vi "Instrument fgv.vi"(7 "Enum":T1(ring), 8 "error in (no error) 2":errorcluster, 10 "WriteCC1":string[](array[string])=[""], 11 "INPUT":T2) -> (0 "error":errorcluster, 2 "WriteCC1 2":string[](array[string]), 3 "output":T2)   [LabVIEW 2025]
uses:
  <vilib>/Instr/_visa.llb/VISA Configure Serial Port (Instr).vi
panel:
  out "error out":errorcluster
  out "Serial Settings:Number of Bytes at Serial Port":u32
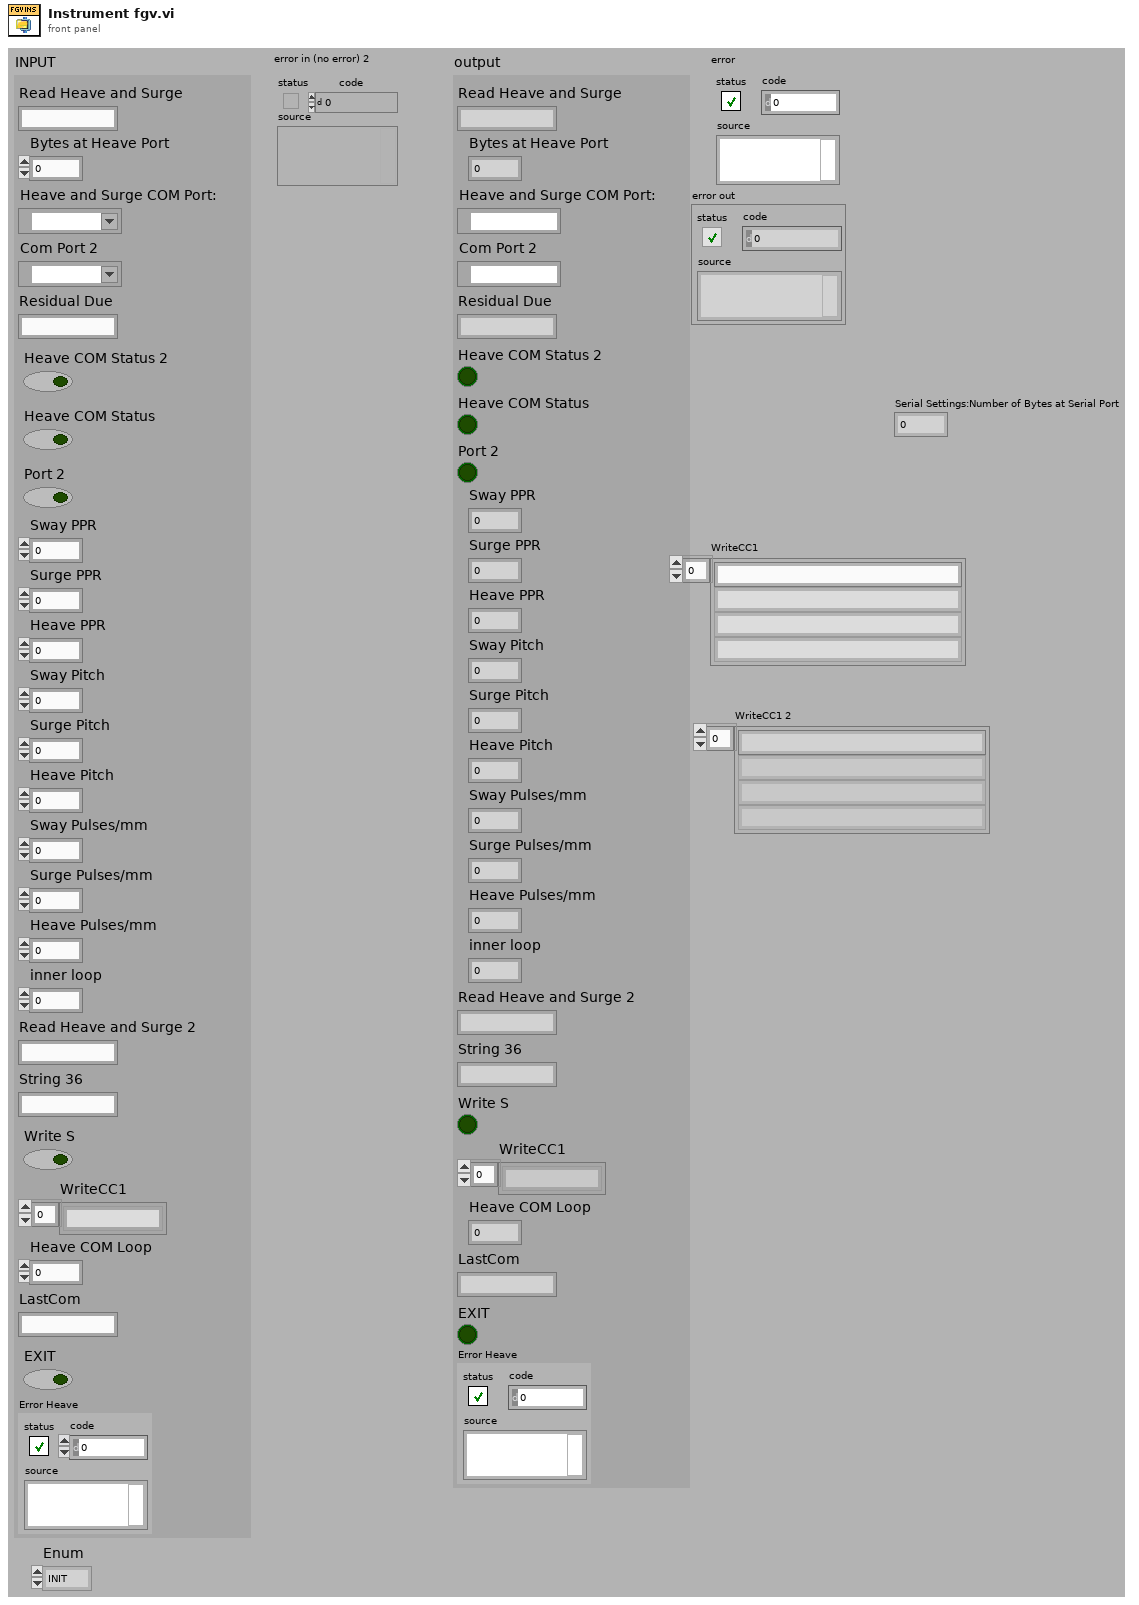
[diagram p1: front panel]
types:
  T1 = enum16{"INIT", "READ", "MANUAL WRITE", "WRITE", "CLOSE", "ERROR INIT"}
  T2 = cluster{"Read Heave and Surge":string, "Bytes at Heave Port":dbl, "Heave and Surge COM Port:":refnum<visa-resource-name>, "Com Port 2":refnum<visa-resource-name>, "Residual Due":string, "Heave COM Status 2":bool, "Heave COM Status":bool, "Port 2":bool, "Sway PPR":dbl, "Surge PPR":dbl, "Heave PPR":dbl, "Sway Pitch":dbl, "Surge Pitch":dbl, "Heave Pitch":dbl, "Sway Pulses/mm":dbl, "Surge Pulses/mm":dbl, "Heave Pulses/mm":dbl, "inner loop":dbl, "Read Heave and Surge 2":string, "String 36":string, "Write S":bool, "WriteCC1":string[], "Heave COM Loop":i32, "LastCom":string, "EXIT":bool, "Error Heave":errorcluster}
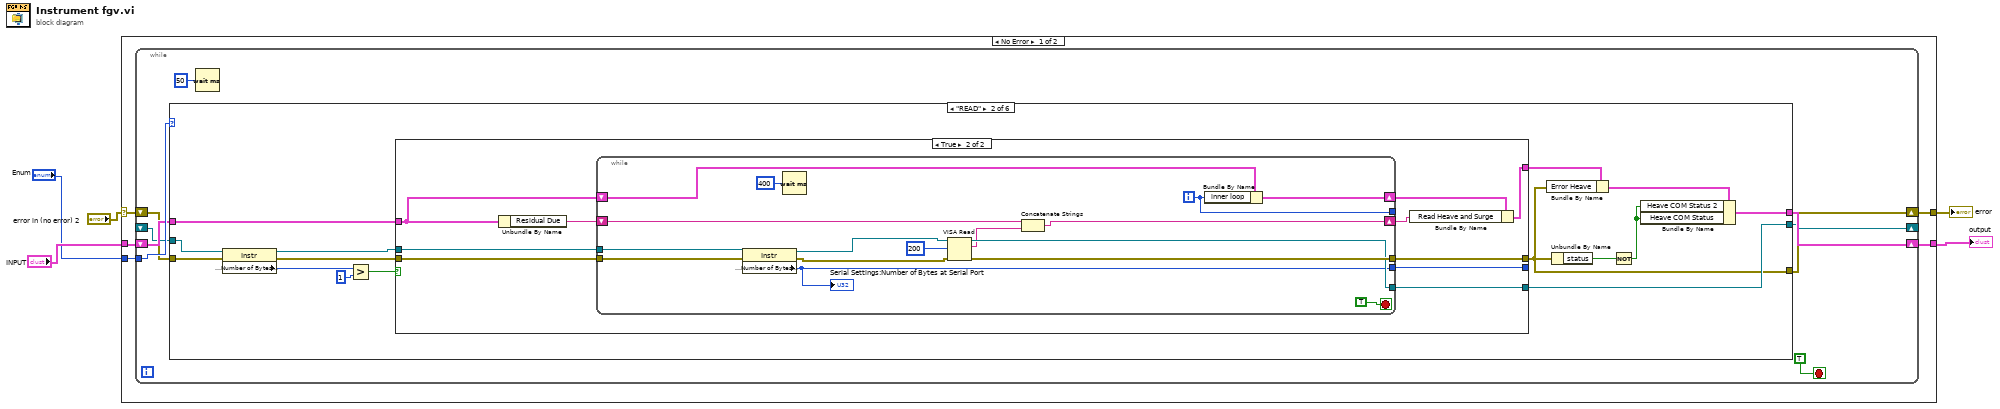
[diagram p0: block diagram]
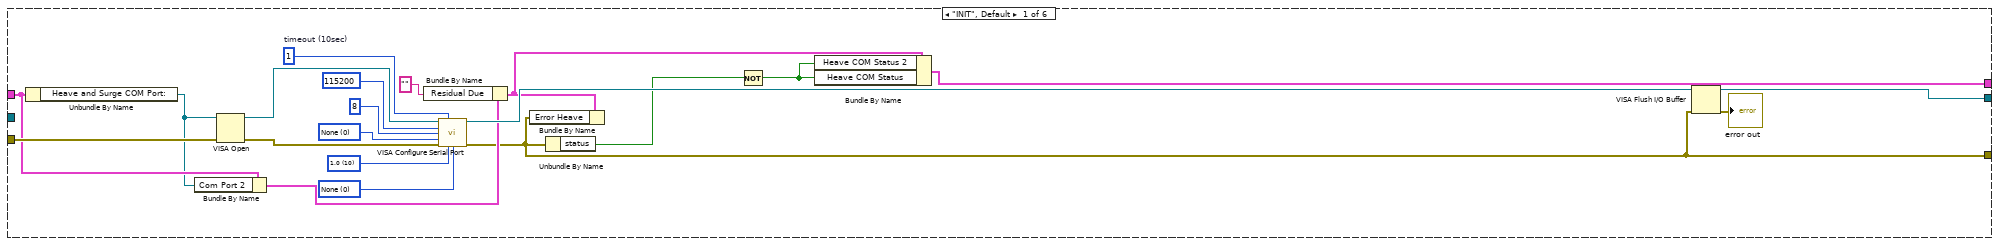
[diagram p2: hidden frame]
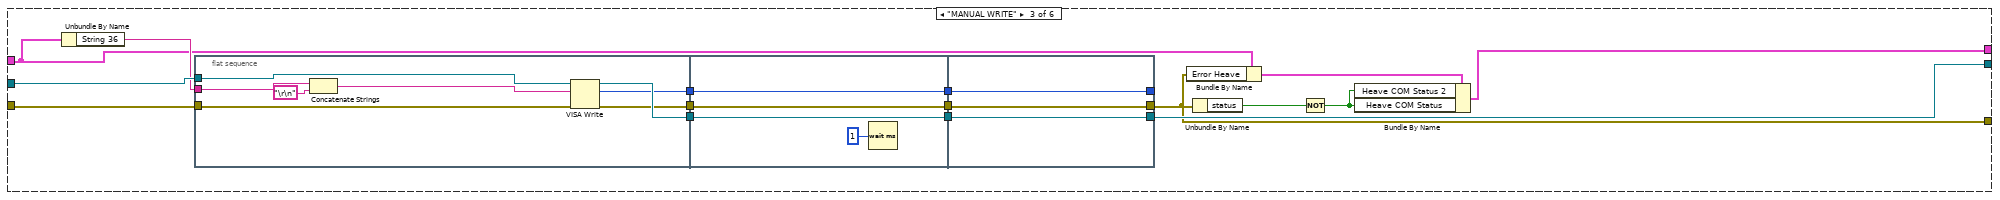
[diagram p4: hidden frame]
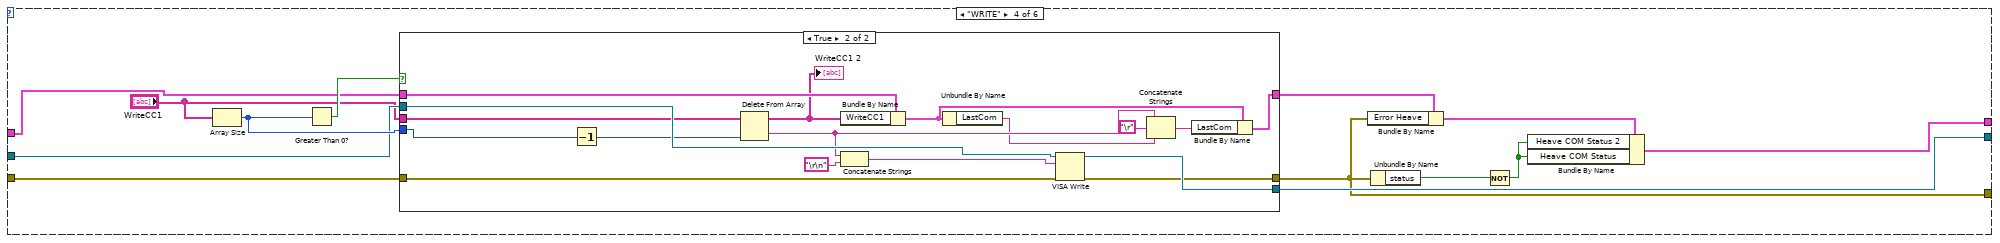
[diagram p5: hidden frame]
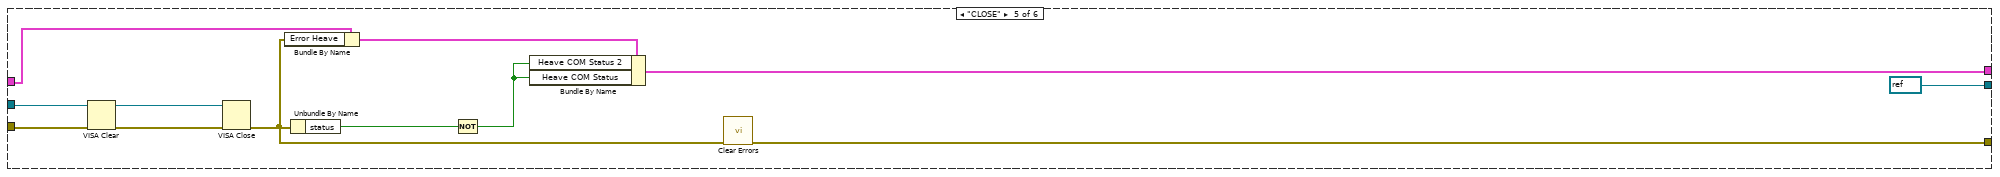
[diagram p7: hidden frame]
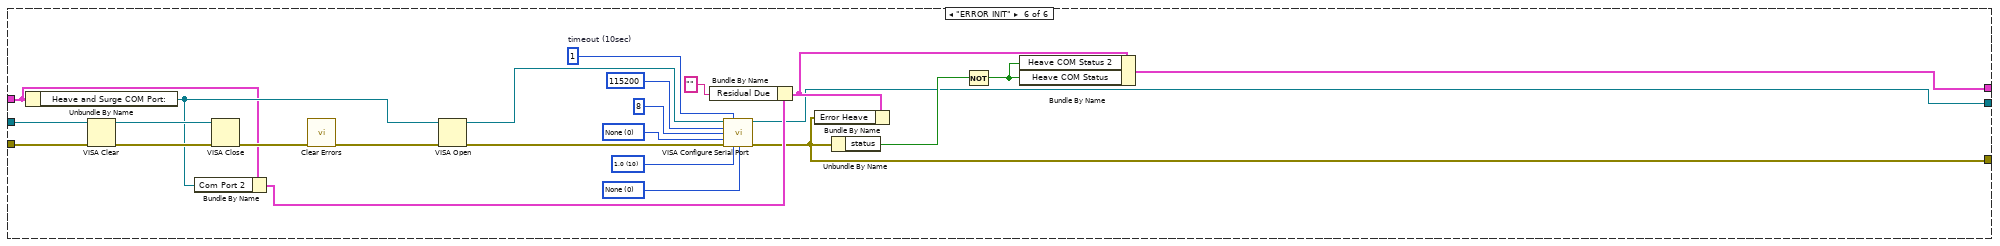
[diagram p8: hidden frame]
diagram:
  n1 = case shown="No Error" "error in (no error) 2" {
    selector: "error in (no error) 2" -> [w9 w185]
    tunnel: [w10 w185] -> w2
    tunnel: "Enum" -> [w8 _]
    tunnel: "INPUT" -> [w7 w186]
    tunnel: [w6 w186] -> w5
    frame No Error {
      n2 = while {
        tunnel: w8 -> [w18]
        shift-right: [w14] -> w10
        shift-left: w9 -> [w15]
        shift-right: [w17] -> w6
        shift-left: w7 -> [w16]
        shift-right: [w13] -> _
        shift-left: _ -> [w12]
        stop <- TRUE ("stop 3") stop-if-true
        n3 = case shown="\"READ\"" w18 {
          tunnel: [w29 w44 w86 w120 w150 w161] -> w17
          tunnel: w16 -> [w25 w48 w88 w123 w151 w165]
          tunnel: w15 -> [w26 w55 w92 w125 w158 w181]
          tunnel: [w21 w41 w87 w119 w156 w163] -> w14
          tunnel: [w22 w43 w93 w124 refnum<visa-resource-name> refnum ("duplicate VISA resource name") w162] -> w13
          tunnel: w12 -> [_ w54 w94 w126 w157 w180]
          frame "INIT", Default {
            w39 = u16 0 items=["None", "XON/XOFF", "RTS/CTS", "XON/XOFF & RTS/CTS", "DTR/DSR", "XON/XOFF & DTR/DSR"] ("flow control (0:none)  2")
            w37 = u16 10 items=["1.0"=10, "1.5"=15, "2.0"=20] ("stop bits 2")
            w36 = u16 0 items=["None", "Odd", "Even", "Mark", "Space"] ("parity 2")
            w34 = u32 1  # timeout (10sec)
            n4 = Unbundle By Name(w25) -> ("Heave and Surge COM Port:"=w23:refnum<visa-resource-name>)
            n5 = Bundle By Name(cluster=w25, "Com Port 2"=w23) -> (w24:T2)
            n6 = VISA Open(error in (no error)=w26, VISA resource name=w23) -> (VISA resource name=w32:refnum<visa-resource-name>, error out=w33:errorcluster)  [unwired: 3 in]
            n7 = Bundle By Name(cluster=w24, "Residual Due"="") -> (w30:T2)
            n8 = call-poly "VISA Configure Serial Port"("VISA resource name"=w32, "timeout (10sec)"=w34, "baud rate (9600)"=u32 115200 ("baud rate  2"), "data bits (8)"=u16 8 ("data bits  2"), "parity (0:none)"=w36, "error in (no error)"=w33, "stop bits (10: 1 bit)"=w37, "flow control (0:none)"=w39) -> ("VISA resource name out"=w31:refnum<visa-resource-name>, "error out"=w21:errorcluster)  [unwired: 6 in]
            n9 = Bundle By Name(cluster=w30, "Error Heave"=w21) -> ()  [unwired: 1 out]
            n10 = Unbundle By Name(w21) -> ("status"=w28:bool)
            n11 = Not(x=w28) -> (.not. x?=w27:bool)
            n12 = Bundle By Name(cluster=w30, "Heave COM Status 2"=w27, "Heave COM Status"=w27) -> (w29:T2)
            n13 = VISA Flush I/O Buffer(VISA resource name=w31, error in (no error)=w21) -> (VISA resource name out=w22:refnum<visa-resource-name>, error out=→"error out":errorcluster)  [unwired: 1 in]
          }
          frame "READ" {
            n14 = property class="Instr"(reference=w54, error in=w55) -> (reference out=w50:refnum<visa-resource-name>, error out=w49:errorcluster, "Serial Settings:Number of Bytes at Serial Port"=w53:u32)
            n15 = Greater?(x=w53, y=u32 1) -> (0:w51:bool)
            n16 = case shown="True" w51 {
              tunnel: w50 -> [w58 w65]
              tunnel: w49 -> [w57 w66]
              tunnel: [w57 w68] -> w41
              tunnel: [w58 w67] -> w43
              tunnel: w48 -> [w56 w64]
              tunnel: [w56 w61] -> w47
              tunnel: [_ w59] -> _
              frame False {
              }
              frame True {
                n17 = Unbundle By Name(w64) -> ("Residual Due"=w63:string)
                n18 = while {
                  tunnel: [w82] -> w68
                  tunnel: [w81] -> w67
                  tunnel: w66 -> [w80]
                  tunnel: w65 -> [w79]
                  tunnel: [w73] -> _
                  shift-right: [w78] -> w60
                  shift-left: w63 -> [w77]
                  shift-right: [w74] -> w62
                  shift-left: w64 -> [w75]
                  tunnel: [w70] -> w59
                  i -> [w73]
                  stop <- TRUE stop-if-true
                  n19 = property class="Instr"(reference=w79, error in=w80) -> (reference out=w84:refnum<visa-resource-name>, error out=w83:errorcluster, "Serial Settings:Number of Bytes at Serial Port"=w70:u32)
                  "Serial Settings:Number of Bytes at Serial Port" <- w70
                  n20 = Wait (ms)(milliseconds to wait=u32 400) -> ()  [unwired: 1 out]
                  n21 = VISA Read(VISA resource name=w84, byte count=u32 200, error in (no error)=w83) -> (VISA resource name out=w81:refnum<visa-resource-name>, read buffer=w76:string, error out=w82:errorcluster)  [unwired: 1 out]
                  n22 = Concatenate Strings(w77, w76) -> (w78:string)
                  n23 = Bundle By Name(cluster=w75, "inner loop"=w73) -> (w74:T2)
                }
                n24 = Bundle By Name(cluster=w62, "Read Heave and Surge"=w60) -> (w61:T2)
              }
            }
            n25 = Bundle By Name(cluster=w47, "Error Heave"=w41) -> (w46:T2)
            n26 = Unbundle By Name(w41) -> ("status"=w45:bool)
            n27 = Not(x=w45) -> (.not. x?=w42:bool)
            n28 = Bundle By Name(cluster=w46, "Heave COM Status 2"=w42, "Heave COM Status"=w42) -> (w44:T2)
          }
          frame "MANUAL WRITE" {
            n29 = Unbundle By Name(w88) -> ("String 36"=w91:string)
            n30 = flat-sequence {
              tunnel: w94 -> [w105]
              tunnel: w92 -> [w104]
              tunnel: w91 -> [w103]
              tunnel: [w108] -> w100
              tunnel: [w107] -> w99
              tunnel: [w106] -> w98
              tunnel: w100 -> [w112]
              tunnel: w99 -> [w111]
              tunnel: w98 -> [w110]
              tunnel: [w112] -> w97
              tunnel: [w111] -> w96
              tunnel: [w110] -> w95
              tunnel: [w113] -> _
              tunnel: [w114] -> w87
              tunnel: [w115] -> w93
              tunnel: w97 -> [w115]
              tunnel: w96 -> [w114]
              tunnel: w95 -> [w113]
              frame #0 {
                n31 = Concatenate Strings(w103, "\r\n") -> (w102:string)
                n32 = VISA Write(VISA resource name=w105, write buffer=w102, error in (no error)=w104) -> (VISA resource name out=w108:refnum<visa-resource-name>, return count=w106:u32, error out=w107:errorcluster)
              }
              frame #1 {
                n33 = Wait (ms)(milliseconds to wait=u32 1) -> ()  [unwired: 1 out]
              }
              frame #2 {
              }
            }
            n34 = Bundle By Name(cluster=w88, "Error Heave"=w87) -> (w90:T2)
            n35 = Unbundle By Name(w87) -> ("status"=w89:bool)
            n36 = Not(x=w89) -> (.not. x?=w85:bool)
            n37 = Bundle By Name(cluster=w90, "Heave COM Status 2"=w85, "Heave COM Status"=w85) -> (w86:T2)
          }
          frame "WRITE" {
            n38 = Array Size(array="WriteCC1") -> (size(s)=w128:i32)
            n39 = Greater Than 0?(x=w128) -> (x > 0?=w127:bool)
            n40 = case shown="True" w127 {
              tunnel: [w131 w141] -> w119
              tunnel: w125 -> [w131 w147]
              tunnel: [w130 w145] -> w124
              tunnel: w126 -> [w130 w146]
              tunnel: "WriteCC1" -> [_ w142]
              tunnel: w128 -> [_ w144]
              tunnel: w123 -> [w129 w138]
              tunnel: [w129 w135] -> w122
              frame False {
              }
              frame True {
                n41 = Decrement(x=w144) -> (x-1=w143:i32)
                n42 = Delete From Array(array=w142, index=w143) -> (deleted portion=w140:string, array with subset deleted=w134:string[])  [unwired: 1 in]
                "WriteCC1 2" <- w134
                n43 = Bundle By Name(cluster=w138, "WriteCC1"=w134) -> (w137:T2)
                n44 = Concatenate Strings(w140, "\r\n") -> (w133:string)
                n45 = Unbundle By Name(w137) -> ("LastCom"=w136:string)
                n46 = VISA Write(VISA resource name=w146, write buffer=w133, error in (no error)=w147) -> (VISA resource name out=w145:refnum<visa-resource-name>, error out=w141:errorcluster)  [unwired: 1 out]
                n47 = Concatenate Strings(w140, "\r", w136) -> (w139:string)
                n48 = Bundle By Name(cluster=w137, "LastCom"=w139) -> (w135:T2)
              }
            }
            n49 = Bundle By Name(cluster=w122, "Error Heave"=w119) -> (w121:T2)
            n50 = Unbundle By Name(w119) -> ("status"=w118:bool)
            n51 = Not(x=w118) -> (.not. x?=w117:bool)
            n52 = Bundle By Name(cluster=w121, "Heave COM Status 2"=w117, "Heave COM Status"=w117) -> (w120:T2)
          }
          frame "CLOSE" {
            n53 = VISA Clear(VISA resource name=w157, error in (no error)=w158) -> (VISA resource name out=w160:refnum<visa-resource-name>, error out=w159:errorcluster)
            n54 = VISA Close(VISA resource name=w160, error in (no error)=w159) -> (error out=w152:errorcluster)
            n55 = Bundle By Name(cluster=w151, "Error Heave"=w152) -> (w155:T2)
            n56 = Unbundle By Name(w152) -> ("status"=w154:bool)
            n57 = Not(x=w154) -> (.not. x?=w153:bool)
            n58 = Bundle By Name(cluster=w155, "Heave COM Status 2"=w153, "Heave COM Status"=w153) -> (w150:T2)
            n59 = call <vilib>:"Clear Errors.vi"("error in (no error)"=w152) -> ("error out"=w156:errorcluster)  [unwired: 5 in, 1 out]
          }
          frame "ERROR INIT" {
            w178 = u16 0 items=["None", "XON/XOFF", "RTS/CTS", "XON/XOFF & RTS/CTS", "DTR/DSR", "XON/XOFF & DTR/DSR"] ("flow control (0:none)  2")
            w176 = u16 10 items=["1.0"=10, "1.5"=15, "2.0"=20] ("stop bits 2")
            w175 = u16 0 items=["None", "Odd", "Even", "Mark", "Space"] ("parity 2")
            w173 = u32 1  # timeout (10sec)
            n60 = Unbundle By Name(w165) -> ("Heave and Surge COM Port:"=w166:refnum<visa-resource-name>)
            n61 = VISA Clear(VISA resource name=w180, error in (no error)=w181) -> (VISA resource name out=w184:refnum<visa-resource-name>, error out=w183:errorcluster)
            n62 = Bundle By Name(cluster=w165, "Com Port 2"=w166) -> (w167:T2)
            n63 = VISA Close(VISA resource name=w184, error in (no error)=w183) -> (error out=w182:errorcluster)
            n64 = call <vilib>:"Clear Errors.vi"("error in (no error)"=w182) -> ("error out"=w164:errorcluster)  [unwired: 5 in, 1 out]
            n65 = VISA Open(error in (no error)=w164, VISA resource name=w166) -> (VISA resource name=w171:refnum<visa-resource-name>, error out=w172:errorcluster)  [unwired: 3 in]
            n66 = Bundle By Name(cluster=w167, "Residual Due"="") -> (w170:T2)
            n67 = call-poly "VISA Configure Serial Port"("VISA resource name"=w171, "timeout (10sec)"=w173, "baud rate (9600)"=u32 115200 ("baud rate  2"), "data bits (8)"=u16 8 ("data bits  2"), "parity (0:none)"=w175, "error in (no error)"=w172, "stop bits (10: 1 bit)"=w176, "flow control (0:none)"=w178) -> ("VISA resource name out"=w162:refnum<visa-resource-name>, "error out"=w163:errorcluster)  [unwired: 6 in]
            n68 = Bundle By Name(cluster=w170, "Error Heave"=w163) -> ()  [unwired: 1 out]
            n69 = Unbundle By Name(w163) -> ("status"=w169:bool)
            n70 = Not(x=w169) -> (.not. x?=w168:bool)
            n71 = Bundle By Name(cluster=w170, "Heave COM Status 2"=w168, "Heave COM Status"=w168) -> (w161:T2)
          }
        }
        n72 = Wait (ms)(milliseconds to wait=u32 50) -> ()  [unwired: 1 out]
      }
    }
    frame Error {
    }
  }
  "output" <- w5
  "error" <- w2
